vi "TempFGV2.vi"(10 "Command":enum16{"Write", "Read"}(ring), 11 "element 3":waveform(dbl)) -> (3 "element 2":waveform(dbl))   [LabVIEW 2015]
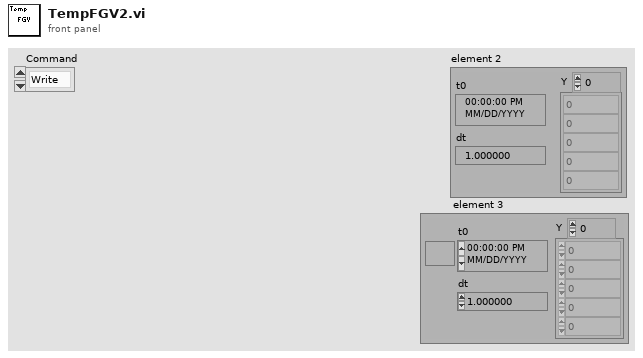
[diagram p1: front panel]
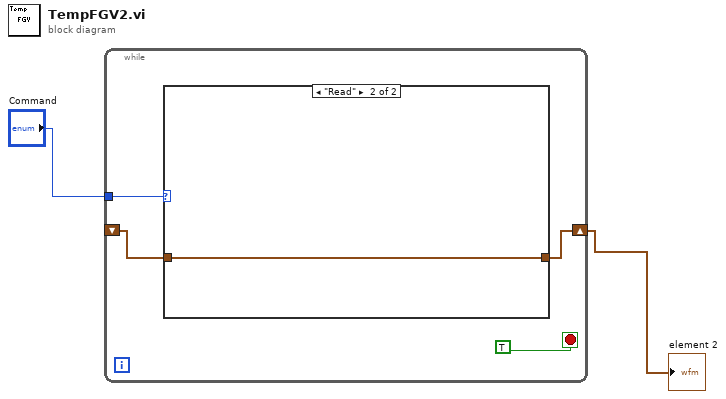
[diagram p0: block diagram]
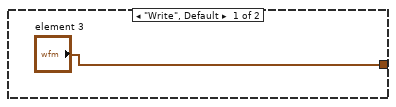
[diagram p2: hidden frame]
diagram:
  n1 = while {
    tunnel: "Command" -> [w6]
    shift-right: [w5] -> w1
    shift-left: _ -> [w3]
    stop <- TRUE stop-if-true
    n2 = case shown="\"Read\"" w6 {
      tunnel: ["element 3" w8] -> w5
      tunnel: w3 -> [_ w8]
      frame "Write", Default {
      }
      frame "Read" {
      }
    }
  }
  "element 2" <- w1
